vi "Publish Group.vi"(8 "error in (no error)":errorcluster, 10 "Group":refnum<class "Group.lvclass">, 11 "RemoteDataService in":refnum<class "RemoteDataService.lvclass">) -> (0 "error out":errorcluster, 3 "RemoteDataService out":refnum<class "RemoteDataService.lvclass">)   [LabVIEW 2020, in "Vecto.lvlib" / "RemoteDataService.lvclass"]
uses:
  RemoteDataService.lvclass
  Group/Group.lvclass
  Publish Group Data.ctl
  lv-protoc/LV-Proto/Message/Message.lvclass
  Group Data Type.ctl
  RemoteDataService.lvclass/RemoteDataService.ctl
  Group/Group.lvclass/Group.ctl
  Group Config/Group Config.lvclass/Group Config.ctl
  Group Config/Group Data Type.vi
  VectoConfig/VectoConfig.lvlib
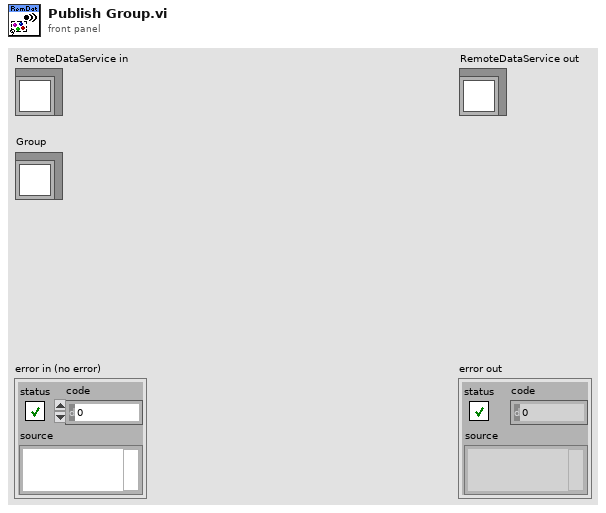
[diagram p1: front panel]
types:
  T1 = typedef "Vecto.lvlib/RemoteDataService.lvclass/Publish Group Data.ctl" = cluster{"Data Msg":refnum<class "Message.lvclass">, "Group Name":string, "Data Type":T2}
  T2 = typedef "VectoConfig.lvlib/Group Data Type.ctl" = enum16{"Double", "String", "Bool"}
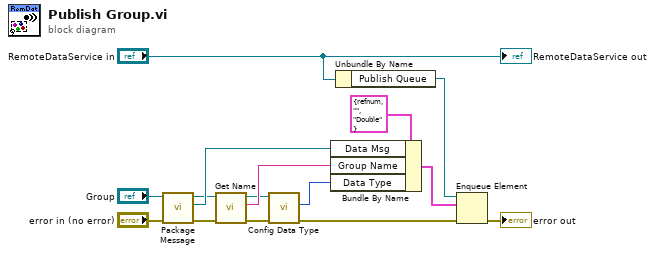
[diagram p0: block diagram]
diagram:
  n1 = call "Package Message.vi"("error in (no error)"="error in (no error)", "Group in"="Group") -> ("error out"=w6:errorcluster, "Data Msg"=w8:refnum<class "Message.lvclass">, "Group out"=w7:refnum<class "Group.lvclass">)  [unwired: 7 in]
  n2 = call "Get Name.vi"("error in (no error)"=w6, "Group in"=w7) -> ("error out"=w3:errorcluster, "Name"=w5:string, "Group out"=w4:refnum<class "Group.lvclass">)  [unwired: 7 in]
  n3 = call "Config Data Type.vi"("error in (no error)"=w3, "Group in"=w4) -> ("error out"=w1:errorcluster, "Group Data Type"=w2:T2)  [unwired: 7 in, 1 out]
  n4 = Bundle By Name(cluster=T1 {"Data Msg"=refnum, "Group Name"="", "Data Type"=enum."Double"} ("event data"), "Data Msg"=w8, "Group Name"=w5, "Data Type"=w2) -> (w12:T1)
  n5 = Unbundle By Name("RemoteDataService in") -> ("Publish Queue"=w14:refnum<queue>)
  n6 = Enqueue Element(queue=w14, element=w12, error in (no error)=w1) -> (error out=→"error out":errorcluster)  [unwired: 1 in, 2 out]
  "RemoteDataService out" <- "RemoteDataService in"
